vi "get_nice_minmax.vi"(10 "Enum":enum16{"min", "max"}(ring), 11 "input":sgl) -> (3 "output":sgl)   [LabVIEW 2020, in "3DPC_SurfacePlot.xctl"]
uses:
  <vilib>/Native 3D Graph/xcontrol/3DPC_SurfacePlot.xctl
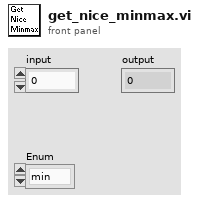
[diagram p1: front panel]
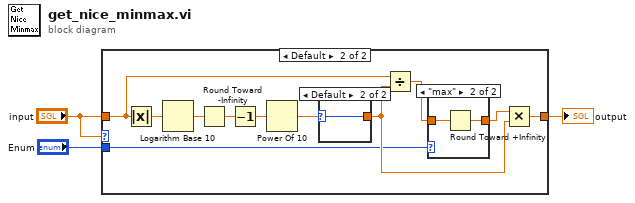
[diagram p0: block diagram]
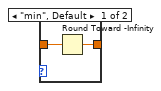
[diagram p3: hidden frame]
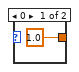
[diagram p4: hidden frame]
diagram:
  n1 = case shown="Default" "input" {
    tunnel: [w4 w12] -> w3
    tunnel: "input" -> [w4 w8]
    tunnel: "Enum" -> [_ w5]
    frame 0 {
    }
    frame Default {
      n2 = Absolute Value(x=w8) -> (abs(x)=w11:sgl)
      n3 = Logarithm Base 10(1:w11) -> (0:w15:sgl)
      n4 = Round Toward -Infinity(1:w15) -> (0:w14:sgl)
      n5 = Decrement(x=w14) -> (x-1=w13:sgl)
      n6 = Power Of 10(x=w13) -> (10^x=w9:sgl)
      n7 = case shown="Default" w9 {
        selector: w9 -> [_ w21]
        tunnel: [sgl 1.0 w21] -> w10
        frame 0 {
        }
        frame Default {
        }
      }
      n8 = Divide(x=w8, y=w10) -> (x/y=w7:sgl)
      n9 = case shown="\"max\"" w5 {
        tunnel: w7 -> [w17 w19]
        tunnel: [w16 w18] -> w6
        frame "min", Default {
          n10 = Round Toward -Infinity(1:w17) -> (0:w16:sgl)
        }
        frame "max" {
          n11 = Round Toward +Infinity(x=w19) -> (ceil(x): smallest int >= x=w18:sgl)
        }
      }
      n12 = Multiply(x=w6, y=w10) -> (x*y=w12:sgl)
    }
  }
  "output" <- w3
